vi "사용자 컨트롤.vi"() -> ()   [LabVIEW 2014]
panel:
  in  "확인 버튼":bool
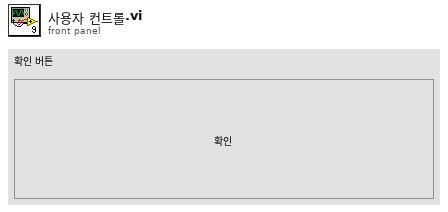
[diagram p1: front panel]
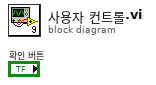
[diagram p0: block diagram]
diagram:
